vi "json Insert I32 - array path.vi"(8 "error in (no error)":errorcluster, 9 "anything":i32, 10 "path":string[](array[string]), 11 "JSON Document in":refnum<class "JSON Document.lvclass">) -> (0 "error out":errorcluster, 3 "JSON Document out":refnum<class "JSON Document.lvclass">)   [LabVIEW 2015, in "JSON Document.lvclass"]
uses:
  JSON Document.lvclass
  json Insert I32 - string path.vi
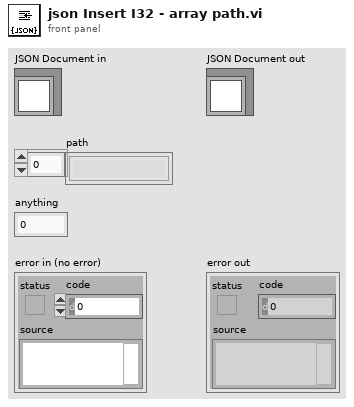
[diagram p1: front panel]
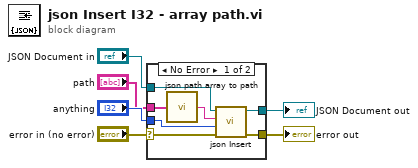
[diagram p0: block diagram]
diagram:
  n1 = case shown="No Error" "error in (no error)" {
    selector: "error in (no error)" -> [w9 w15]
    tunnel: [w8 w15] -> w5
    tunnel: [w7 w14] -> w3
    tunnel: "JSON Document in" -> [w12 w14]
    tunnel: "anything" -> [w10 _]
    tunnel: "path" -> [w11 _]
    frame No Error {
      n2 = call "json path array to path.vi"("path"=w11) -> ("String"=w13:string)
      n3 = call-poly "json Insert.vi"("error in (no error)"=w9, "anything"=w10, "path"=w13, "JSON Document in"=w12) -> ("error out"=w8:errorcluster, "JSON Document out"=w7:refnum<class "JSON Document.lvclass">)  [unwired: 6 in]
    }
    frame Error {
    }
  }
  "error out" <- w5
  "JSON Document out" <- w3
